vi "I2C Change CS.vi"(8 "error in (no error)":errorcluster, 10 "configOptions":u32, 11 "handle":u32) -> (0 "error out":errorcluster, 2 "function return":u32, 3 "handle out":u32)   [LabVIEW 2024, in "libMPSSE-I2C.lvlib"]
doc: "FTDI_API FT_STATUS SPI_ChangeCS(FT_HANDLE handle, uint32 configOptions);"
uses:
  libMPSSE-I2C.lvlib
  libmpsse.dll
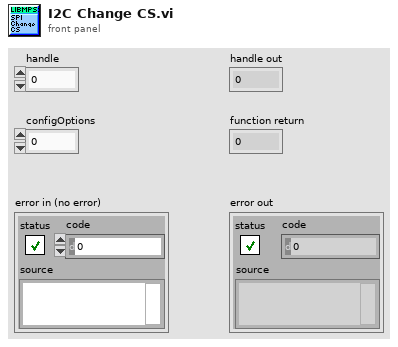
[diagram p1: front panel]
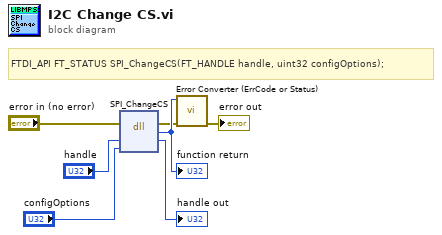
[diagram p0: block diagram]
diagram:
  # "FTDI_API FT_STATUS SPI_ChangeCS(FT_HANDLE handle, uint32 configOptions);"
  n1 = dll-call lib="C:/Workspace/sm_6576_001_RIB_Sequencer/I2C/libmpsse.dll" fn="SPI_ChangeCS"(error in="error in (no error)", "handle"="handle", "configOptions"="configOptions") -> (error out=w2:errorcluster, "return type"=w7:u32, "handle"=→"handle out":u32)  [unwired: 3 in, 1 out]
  "function return" <- w7
  n2 = call "Error Converter (ErrCode or Status).vi"("error in (no error)"=w2, "error code"=w7) -> ("error out"=→"error out":errorcluster)  [unwired: 9 in]
